vi "Set UI GPU Done.vi"(8 "error in (no error)":errorcluster, 10 "GPU Done":bool, 11 "Application Manager in":refnum<class "Application Manager.lvclass">) -> (0 "error out":errorcluster, 3 "Application Manager out":refnum<class "Application Manager.lvclass">)   [LabVIEW 2020, in "Application Manager.lvlib" / "Application Manager.lvclass"]
uses:
  Application Manager.lvclass
  Application Manager.lvclass/Application Manager.ctl
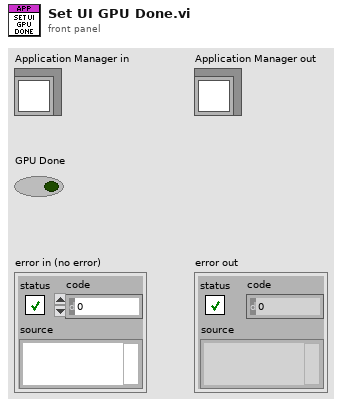
[diagram p1: front panel]
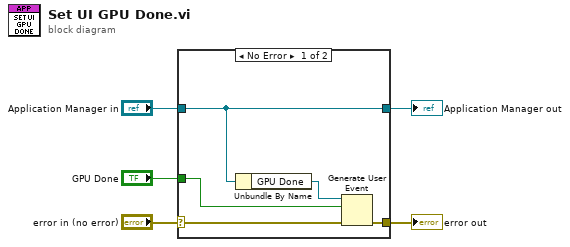
[diagram p0: block diagram]
diagram:
  n1 = case shown="No Error" "error in (no error)" {
    selector: "error in (no error)" -> [w10 w12]
    tunnel: [w9 w12] -> w4
    tunnel: [w7 w11] -> w2
    tunnel: "Application Manager in" -> [w7 w11]
    tunnel: "GPU Done" -> [w8 _]
    frame No Error {
      n2 = Unbundle By Name(w7) -> ("GPU Done"=w6:refnum<user-event>)
      n3 = Generate User Event(user event=w6, event data cluster=w8, error in=w10) -> (error out=w9:errorcluster)  [unwired: 1 in, 1 out]
    }
    frame Error {
    }
  }
  "error out" <- w4
  "Application Manager out" <- w2
